vi "Tree Bookmark ID.vi"(8 "Error In":errorcluster, 10 "Bookmarks":T1[](array[typedef]), 11 "Tag":string) -> (0 "Error Out":errorcluster, 2 "Path":path, 3 "Bookmark ID":u32)   [LabVIEW 2017, in "Bookmark Manager.lvlib"]
uses:
  Bookmark Manager.lvlib
  Controls/VI Bookmark.ctl
  Controls/VI Information.ctl
  Controls/Application Information.ctl
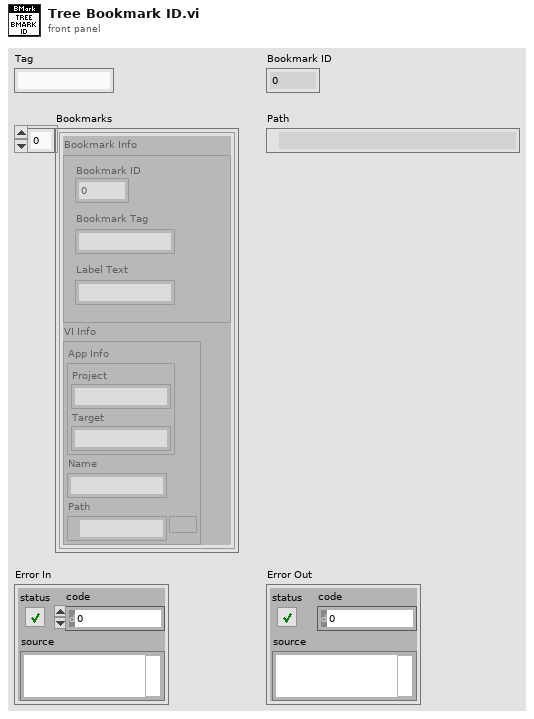
[diagram p1: front panel]
types:
  T1 = typedef "Bookmark Manager.lvlib/VI Bookmark.ctl" = cluster{"Bookmark Info":cluster{"Bookmark ID":u32, "Bookmark Tag":string, "Label Text":string}, "VI Info":T2}
  T2 = typedef "Bookmark Manager.lvlib/VI Information.ctl" = cluster{"App Info":T3, "Name":string, "Path":path}
  T3 = typedef "Bookmark Manager.lvlib/Application Information.ctl" = cluster{"Project":string, "Target":string}
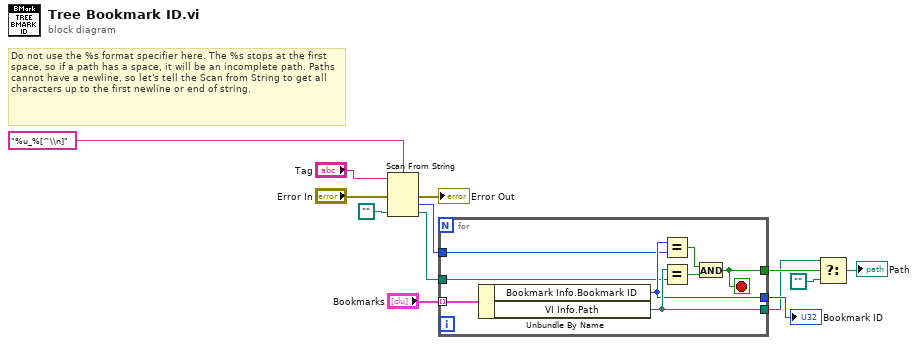
[diagram p0: block diagram]
diagram:
  # "Do not use the %s format specifier here. The %s stops at the first space, so if a path has a space, it will be an incomplete path. Paths cannot have a newline, so let's tell the Scan from String to get all characters up to the first newline or end of string."
  n1 = Scan From String(format string="%u_%[^\\n]", input string="Tag", error in="Error In", default 2=path "") -> (error out=→"Error Out":errorcluster, output 1=w1:u32, output 2=w2:path)  [unwired: 2 in, 2 out]
  n2 = for {
    tunnel: "Bookmarks" -> [w21] mode=indexing
    tunnel: [w18] -> w12
    tunnel: [w17] -> w11
    tunnel: [w19] -> w10
    tunnel: w1 -> [w15]
    tunnel: w2 -> [w14]
    stop <- w17 stop-if-true
    n3 = Unbundle By Name(w21) -> ("Bookmark Info.Bookmark ID"=w18:u32, "VI Info.Path"=w19:path)
    n4 = Equal?(x=w18, y=w15) -> (x = y?=w16:bool)
    n5 = Equal?(x=w19, y=w14) -> (x = y?=w20:bool)
    n6 = And(x=w16, y=w20) -> (x .and. y?=w17:bool)
  }
  "Bookmark ID" <- w12
  n7 = Select(t=w10, s=w11, f=path "") -> (s? t:f=→"Path":path)
